vi "PLQY by corrected.vi"() -> ()   [LabVIEW 2018]
uses:
  <vilib>/Utility/file.llb/Read Delimited Spreadsheet (DBL).vi
  <vilib>/Utility/file.llb/Write Delimited Spreadsheet (DBL).vi
panel:
  out "XY Graph":cluster{"Y":dbl[], "Y":dbl[]}[](graph)
  in  "Sample name":string
  out "PL begin\n wavelength":dbl
  out "PL end \nwavelength":dbl
  in  "OK Button":bool
  in  "Lamp on-- No doule laser on the right\nLamp off- have doule laser on the right\nsuch as 450nm laser, 900nm":bool=TRUE
  out "PL end":dbl
  out "PL begin":dbl
  out "Laser end":dbl
  out "Laser begin":dbl
  in  "Stop":bool
  in  "Begin to calculate":bool
  out "XY Graph 2":cluster{"Y":dbl[], "Y":dbl[]}[](graph) caption="XY图"
  in  "Dichroic ratio":dbl=1.0
  out "PLQY":dbl[](array[numeric]) format="%#_3g"
  in  "file path (dialog if empty) 4":path caption="Reference"
  in  "file path (sample) 3":path caption="Sample"
  in  "file path (blank) 2":path caption="Blank"
  # "2. Press run"
  # "3. Begin to calculate"
  # "1. select blank, sample and reference files"
  # "The converted files will be in the data folder,\nname it by yourself. If there is no name, a file \nwith real time will also be created in the folder."
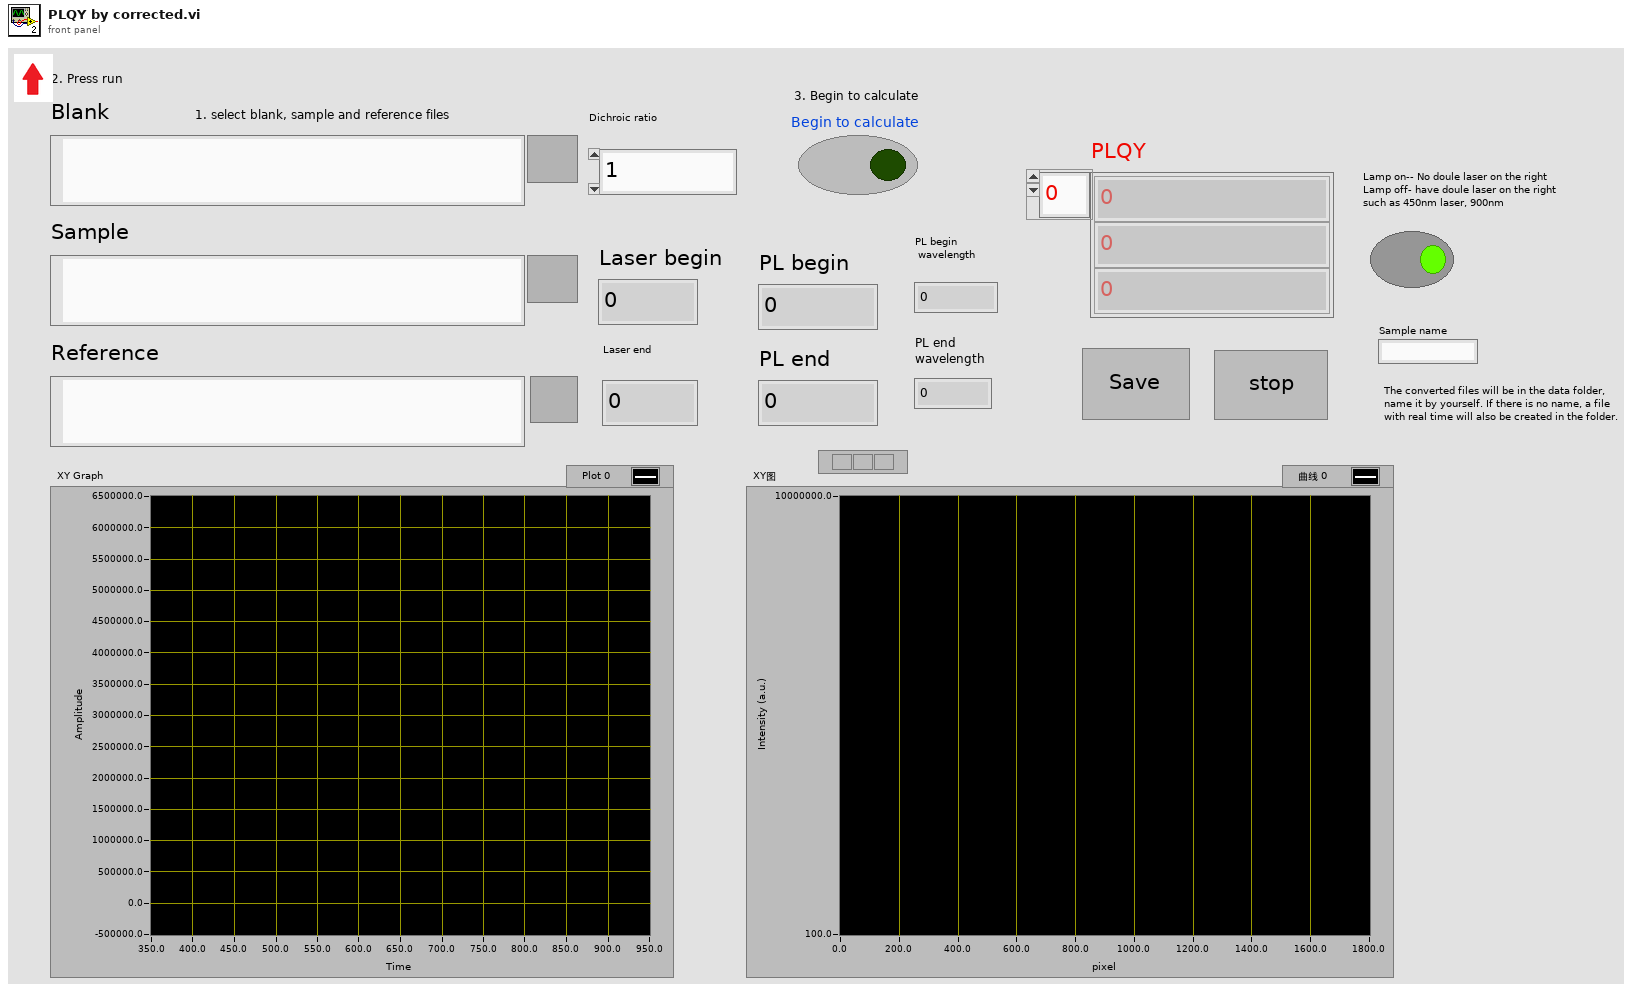
[diagram p1: front panel]
types:
  T1 = typedef "LVCursorListTypeDef.ctl" = cluster{"Name":string, "Color":u32, "Style":u8, "Point Style":u8, "Name Visible":bool, "Allow Drag":bool, "Cursor Mode":u32, "Plot":i32, "Index":i32, "Position":cluster{"X":dbl, "Y":dbl}, "X Scale":u32, "Y Scale":u32, "Watch Plots":i32[], "Watch All Plots":bool, "Plot Area":i32, "Label Offset":cluster{"X":dbl, "Y":dbl}}[]
  T2 = cluster{"Name":string, "Color":u32, "Style":u8, "Point Style":u8, "Name Visible":bool, "Allow Drag":bool, "Cursor Mode":u32, "Plot":i32, "Index":i32, "Position":cluster{"X":dbl, "Y":dbl}, "X Scale":u32, "Y Scale":u32, "Watch Plots":i32[], "Watch All Plots":bool, "Plot Area":i32, "Label Offset":cluster{"X":dbl, "Y":dbl}}
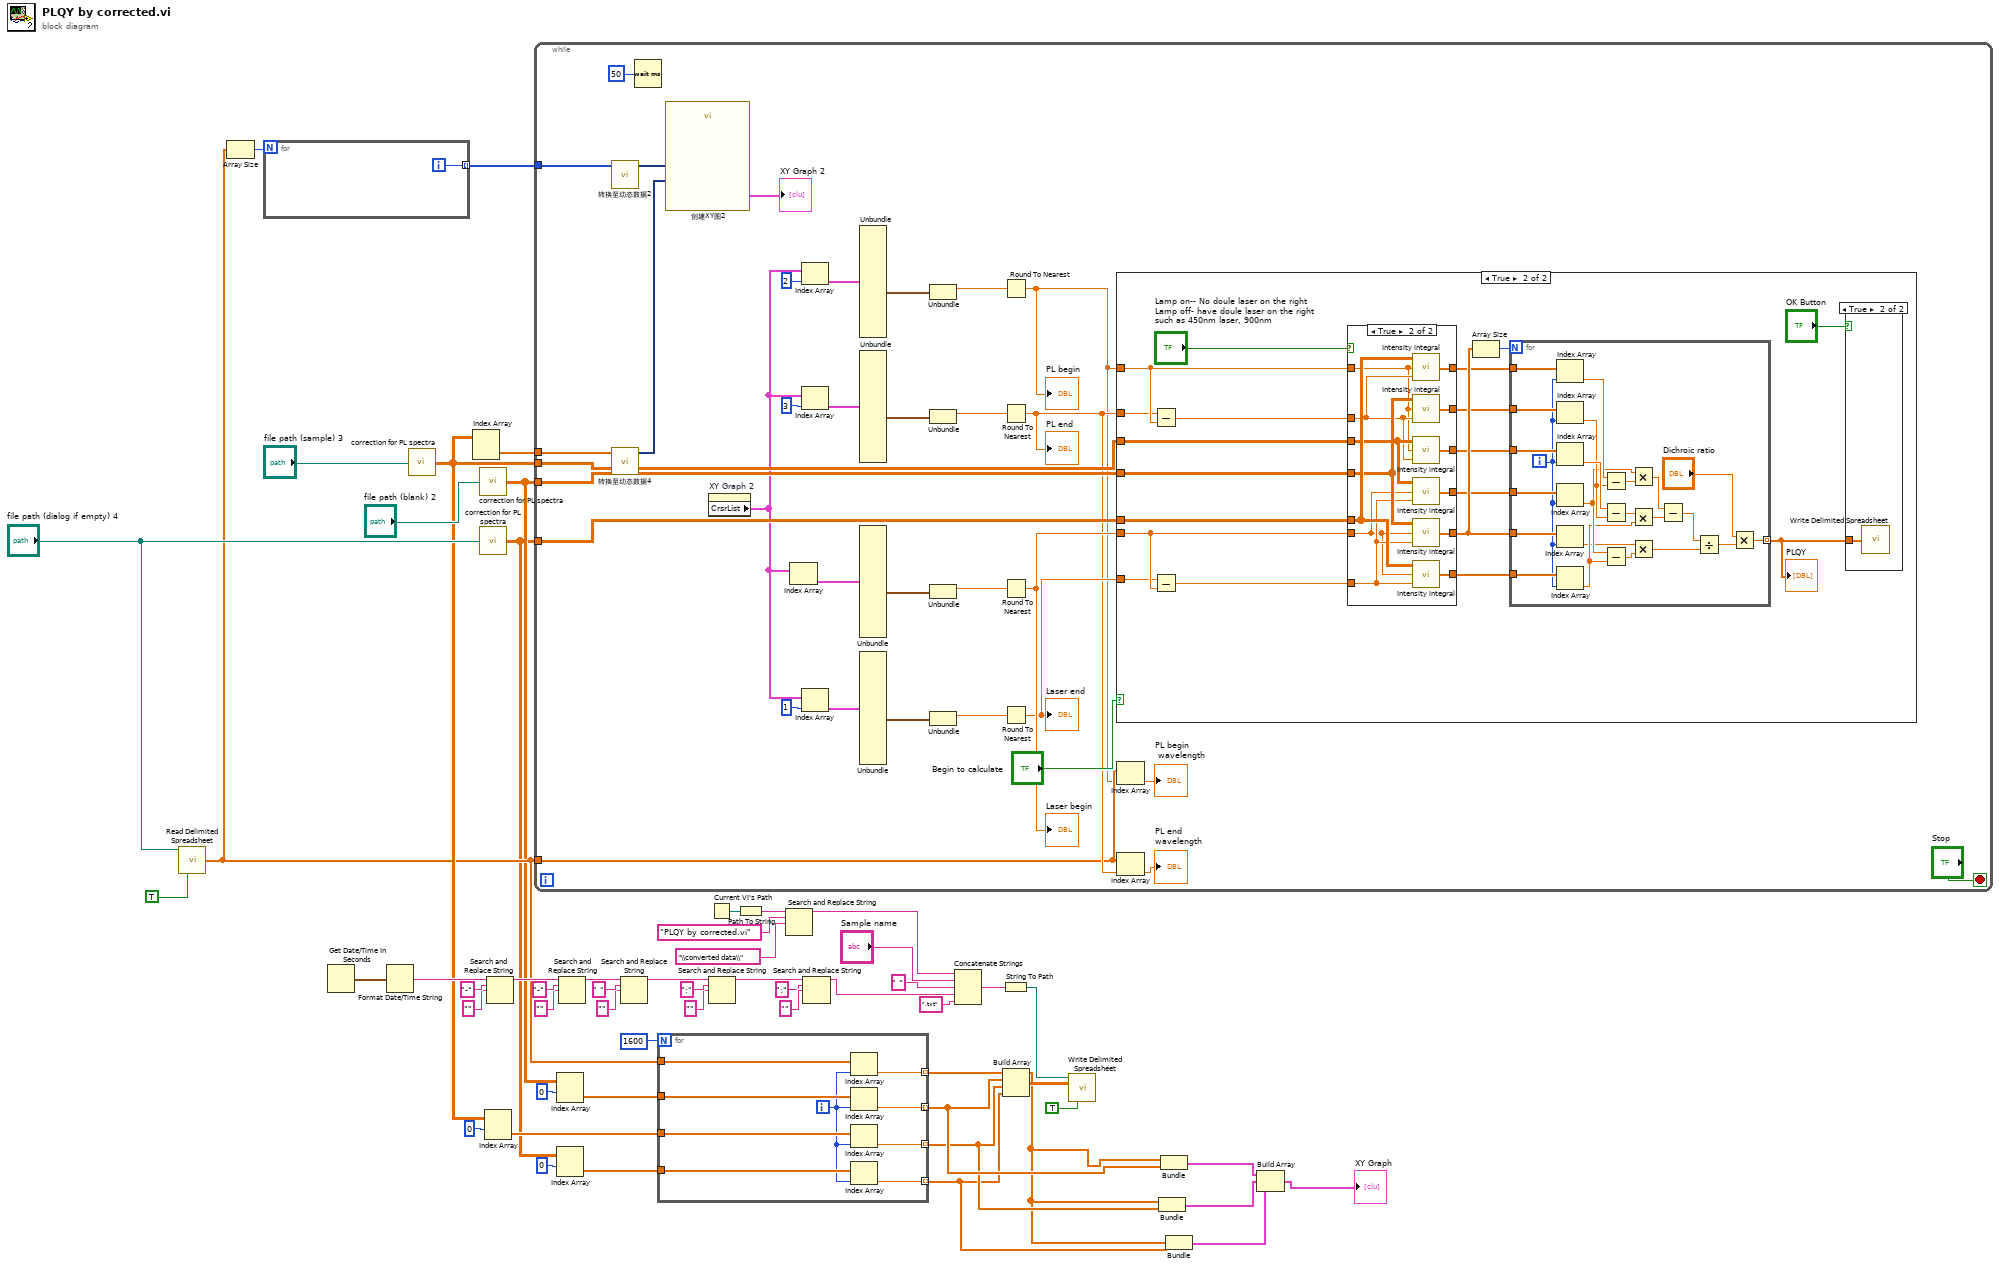
[diagram p0: block diagram]
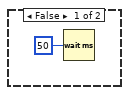
[diagram p2: hidden frame]
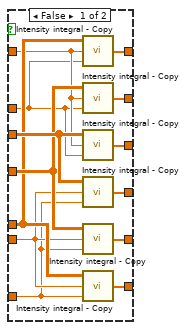
[diagram p4: hidden frame]
diagram:
  n1 = call-poly <vilib>:"Read Delimited Spreadsheet.vi"("file path (dialog if empty)"="file path (dialog if empty) 4", "transpose? (F)"=TRUE) -> ("first row"=w18:dbl[])  [unwired: 8 in, 5 out]
  n2 = Array Size(array=w18) -> (size(s)=w50:i32)
  n3 = for {
    N: w50 -> [_]
    tunnel: [w56] -> w49 mode=indexing
    i -> [w56]
  }
  n4 = Get Date/Time In Seconds() -> (seconds since 1Jan1904=w44:timestamp)
  n5 = Format Date/Time String(seconds (now)=w44) -> (date/time string=w39:string)  [unwired: 2 in]
  n6 = call "correction for PL spectra.vi"("file path (dialog if empty) 2"="file path (sample) 3") -> ("数组 2"=w20:dbl[][])
  n7 = Index Array(array=w20) -> (element=w51:dbl[])  [unwired: 2 in]
  n8 = call "correction for PL spectra.vi"("file path (dialog if empty) 2"="file path (blank) 2") -> ("数组 2"=w15:dbl[][])
  n9 = call "correction for PL spectra.vi"("file path (dialog if empty) 2"="file path (dialog if empty) 4") -> ("数组 2"=w12:dbl[][])
  n10 = Index Array(array=w20, index (row)=0) -> (element=w17:dbl[])  [unwired: 1 in]
  n11 = Search and Replace String(input string=w39, search string="-", replace string="" ("replace string (\"\")")) -> (result string=w38:string)  [unwired: 5 in, 3 out]
  n12 = while {
    tunnel: w12 -> [w90]
    tunnel: w18 -> [w59]
    tunnel: w15 -> [w87]
    tunnel: w20 -> [w86]
    tunnel: w51 -> [w85]
    tunnel: w49 -> [w62]
    stop <- "Stop" stop-if-true
    n13 = call "转换至动态数据2"("Array"=w62) -> ("Dynamic Data Type"=w88:dynamicdata)  [unwired: 3 in]
    n14 = call "转换至动态数据4"("Array"=w85) -> ("Dynamic Data Type"=w84:dynamicdata)  [unwired: 3 in]
    n15 = Wait (ms)(milliseconds to wait=u32 50 ("等待时间（毫秒）")) -> ()  [unwired: 1 out]
    n16 = call "创建XY图2"("Y Input"=w84, "X Input"=w88) -> ("XY Graph"=→"XY Graph 2":cluster{"X":dbl[], "Y":dbl[]}[])  [unwired: 8 in, 1 out]
    n17 = property on="XY Graph 2" class="XYGraph (strict)"() -> ("CrsrList"=w77:T1)  [unwired: 2 in, 2 out]
    n18 = Index Array(array=w77) -> (element=w76:T2)  [unwired: 1 in]
    n19 = Index Array(array=w77, index=2 ("索引")) -> (element=w74:T2)
    n20 = Index Array(array=w77, index=3 ("索引")) -> (element=w73:T2)
    n21 = Index Array(array=w77, index=1 ("索引")) -> (element=w75:T2)
    n22 = Unbundle(w74) -> ("Position"=w70:cluster{"X":dbl, "Y":dbl})  [unwired: 15 out]
    n23 = Unbundle(w73) -> ("Position"=w69:cluster{"X":dbl, "Y":dbl})  [unwired: 15 out]
    n24 = Unbundle(w76) -> ("Position"=w72:cluster{"X":dbl, "Y":dbl})  [unwired: 15 out]
    n25 = Unbundle(w75) -> ("Position"=w71:cluster{"X":dbl, "Y":dbl})  [unwired: 15 out]
    n26 = Unbundle(w70) -> ("X"=w66:dbl)  [unwired: 1 out]
    n27 = Unbundle(w69) -> ("X"=w65:dbl)  [unwired: 1 out]
    n28 = Unbundle(w72) -> ("X"=w68:dbl)  [unwired: 1 out]
    n29 = Unbundle(w71) -> ("X"=w67:dbl)  [unwired: 1 out]
    n30 = Round To Nearest(number=w66) -> (nearest integer value=w58:dbl)
    "PL begin" <- w58
    n31 = Round To Nearest(number=w65) -> (nearest integer value=w61:dbl)
    "PL end" <- w61
    n32 = Round To Nearest(number=w68) -> (nearest integer value=w64:dbl)
    "Laser begin" <- w64
    n33 = Round To Nearest(number=w67) -> (nearest integer value=w63:dbl)
    "Laser end" <- w63
    n34 = case shown="True" "Begin to calculate" {
      tunnel: w90 -> [_ w110]
      tunnel: w87 -> [_ w102]
      tunnel: w86 -> [_ w101]
      tunnel: w64 -> [_ w98]
      tunnel: w63 -> [_ w97]
      tunnel: w58 -> [_ w96]
      tunnel: w61 -> [_ w95]
      frame False {
        n35 = Wait (ms)(milliseconds to wait=u32 50 ("等待时间（毫秒）")) -> ()  [unwired: 1 out]
      }
      frame True {
        n36 = Subtract(x=w95, y=w96) -> (x-y=w99:dbl)
        n37 = Subtract(x=w97, y=w98) -> (x-y=w100:dbl)
        n38 = case shown="True" "Lamp on-- No doule laser on the right\nLamp off- have doule laser on the right\nsuch as 450nm laser, 900nm" {
          tunnel: w110 -> [w116 w137]
          tunnel: [w121 w136] -> w108
          tunnel: [w123 w135] -> w107
          tunnel: [w122 w134] -> w106
          tunnel: [w124 w133] -> w105
          tunnel: [w119 w132] -> w104
          tunnel: [w120 w131] -> w103
          tunnel: w102 -> [w117 w130]
          tunnel: w101 -> [w118 w129]
          tunnel: w100 -> [w112 w128]
          tunnel: w99 -> [w114 w127]
          tunnel: w98 -> [w113 w126]
          tunnel: w96 -> [w115 w125]
          frame False {
            n39 = call "Intensity integral - Copy.vi"("width"=w114, "begin"=w115, "数组"=w116) -> ("数组 2"=w120:dbl[])
            n40 = call "Intensity integral - Copy.vi"("width"=w114, "begin"=w115, "数组"=w117) -> ("数组 2"=w123:dbl[])
            n41 = call "Intensity integral - Copy.vi"("width"=w114, "begin"=w115, "数组"=w118) -> ("数组 2"=w124:dbl[])
            n42 = call "Intensity integral - Copy.vi"("width"=w112, "begin"=w113, "数组"=w118) -> ("数组 2"=w122:dbl[])
            n43 = call "Intensity integral - Copy.vi"("width"=w112, "begin"=w113, "数组"=w117) -> ("数组 2"=w121:dbl[])
            n44 = call "Intensity integral - Copy.vi"("width"=w112, "begin"=w113, "数组"=w116) -> ("数组 2"=w119:dbl[])
          }
          frame True {
            n45 = call "Intensity integral.vi"("width"=w127, "begin"=w125, "数组"=w137) -> ("数组 2"=w131:dbl[])
            n46 = call "Intensity integral.vi"("width"=w127, "begin"=w125, "数组"=w130) -> ("数组 2"=w135:dbl[])
            n47 = call "Intensity integral.vi"("width"=w127, "begin"=w125, "数组"=w129) -> ("数组 2"=w133:dbl[])
            n48 = call "Intensity integral.vi"("width"=w128, "begin"=w126, "数组"=w129) -> ("数组 2"=w134:dbl[])
            n49 = call "Intensity integral.vi"("width"=w128, "begin"=w126, "数组"=w130) -> ("数组 2"=w136:dbl[])
            n50 = call "Intensity integral.vi"("width"=w128, "begin"=w126, "数组"=w137) -> ("数组 2"=w132:dbl[])
          }
        }
        n51 = Array Size(array=w108) -> (size(s)=w109:i32)
        n52 = for {
          N: w109 -> [_]
          tunnel: w108 -> [w160]
          tunnel: w107 -> [w159]
          tunnel: w106 -> [w158]
          tunnel: w105 -> [w157]
          tunnel: w104 -> [w156]
          tunnel: w103 -> [w155]
          tunnel: [w139] -> w93 mode=indexing
          i -> [w154]
          n53 = Index Array(array=w155, index=w154) -> (element=w153:dbl)
          n54 = Index Array(array=w159, index=w154) -> (element=w151:dbl)
          n55 = Index Array(array=w157, index=w154) -> (element=w152:dbl)
          n56 = Index Array(array=w158, index=w154) -> (element=w148:dbl)
          n57 = Index Array(array=w160, index=w154) -> (element=w145:dbl)
          n58 = Index Array(array=w156, index=w154) -> (element=w147:dbl)
          n59 = Subtract(x=w153, y=w151) -> (x-y=w150:dbl)
          n60 = Subtract(x=w152, y=w151) -> (x-y=w149:dbl)
          n61 = Subtract(x=w148, y=w147) -> (x-y=w146:dbl)
          n62 = Multiply(x=w148, y=w150) -> (x*y=w144:dbl)
          n63 = Multiply(x=w149, y=w147) -> (x*y=w143:dbl)
          n64 = Multiply(x=w145, y=w146) -> (x*y=w141:dbl)
          n65 = Subtract(x=w144, y=w143) -> (x-y=w142:dbl)
          n66 = Divide(x=w142, y=w141) -> (x/y=w140:dbl)
          n67 = Multiply(x="Dichroic ratio", y=w140) -> (x*y=w139:dbl)
        }
        "PLQY" <- w93
        n68 = case shown="True" "OK Button" {
          tunnel: w93 -> [_ w111]
          frame False {
          }
          frame True {
            n69 = call-poly <vilib>:"Write Delimited Spreadsheet.vi"("1D data"=w111) -> ()  [unwired: 13 in, 2 out]
          }
        }
      }
    }
    n70 = Index Array(array=w59, index=w58) -> (element=→"PL begin\n wavelength":dbl)
    n71 = Index Array(array=w59, index=w61) -> (element=→"PL end \nwavelength":dbl)
  }
  n72 = Index Array(array=w15, index (row)=0) -> (element=w14:dbl[])  [unwired: 1 in]
  n73 = Index Array(array=w12, index (row)=0) -> (element=w11:dbl[])  [unwired: 1 in]
  n74 = Search and Replace String(input string=w38, search string="-", replace string="" ("replace string (\"\")")) -> (result string=w35:string)  [unwired: 5 in, 3 out]
  n75 = Search and Replace String(input string=w35, search string=" ", replace string="" ("replace string (\"\")")) -> (result string=w31:string)  [unwired: 5 in, 3 out]
  n76 = for {
    N: 1600 -> [_]
    tunnel: w18 -> [w169]
    tunnel: w17 -> [w168]
    tunnel: w14 -> [w167]
    tunnel: w11 -> [w166]
    tunnel: [w164] -> w6 mode=indexing
    tunnel: [w163] -> w8 mode=indexing
    tunnel: [w162] -> w7 mode=indexing
    tunnel: [w161] -> w5 mode=indexing
    i -> [w165]
    n77 = Index Array(array=w169, index=w165) -> (element=w164:dbl)
    n78 = Index Array(array=w167, index=w165) -> (element=w163:dbl)
    n79 = Index Array(array=w168, index=w165) -> (element=w162:dbl)
    n80 = Index Array(array=w166, index=w165) -> (element=w161:dbl)
  }
  n81 = Current VI's Path() -> (path=w48:path)
  n82 = Search and Replace String(input string=w31, search string=":", replace string="" ("replace string (\"\")")) -> (result string=w30:string)  [unwired: 5 in, 3 out]
  n83 = Path To String(path=w48) -> (string=w47:string)
  n84 = Search and Replace String(input string=w47, search string="PLQY by corrected.vi", replace string="\\converted data\\" ("replace string (\"\")")) -> (result string=w28:string)  [unwired: 5 in, 3 out]
  n85 = Search and Replace String(input string=w30, search string=":", replace string="" ("replace string (\"\")")) -> (result string=w25:string)  [unwired: 5 in, 3 out]
  n86 = Concatenate Strings(w28, "Sample name", " " ("string"), w25, ".txt" ("string")) -> (w23:string)
  n87 = String To Path(string=w23) -> (path=w22:path)
  n88 = Build Array(w6, w8, w7, w5) -> (w10:dbl[][])
  n89 = call-poly <vilib>:"Write Delimited Spreadsheet.vi"("file path (dialog if empty)"=w22, "2D data"=w10, "transpose? (no:F)"=TRUE) -> ()  [unwired: 11 in, 2 out]
  n90 = Bundle(w6, w7) -> (w3:cluster{dbl[], dbl[]})  [unwired: 1 in]
  n91 = Bundle(w6, w8) -> (w4:cluster{dbl[], dbl[]})  [unwired: 1 in]
  n92 = Bundle(w6, w5) -> (w2:cluster{dbl[], dbl[]})  [unwired: 1 in]
  n93 = Build Array(w4, w3, w2) -> (→"XY Graph":cluster{dbl[], dbl[]}[])
